vi "dfd_Check Num of Chan.vi"(7 "init in":bool, 8 "error in (no error)":errorcluster, 11 "#ch in":i32) -> (0 "error out":errorcluster, 3 "#ch out":i32, 5 "init out":bool)   [LabVIEW 2017, in "NI_DigFilter_Process.lvlib"]
uses:
  <vilib>/addons/Digital Filter Design/NI_DigFilter_Process.lvlib
  <vilib>/addons/Digital Filter Design/_Misc.llb/dfd_Error Handlers (Single).vi
  <vilib>/addons/Digital Filter Design/NI_DigFilterLicensed.lvlib
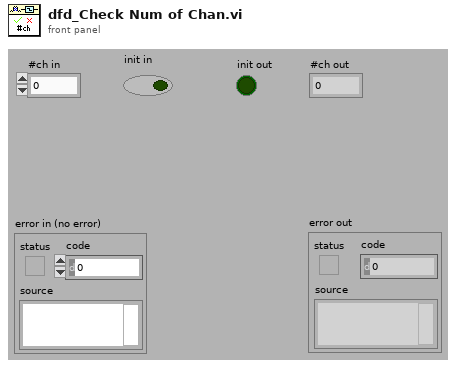
[diagram p1: front panel]
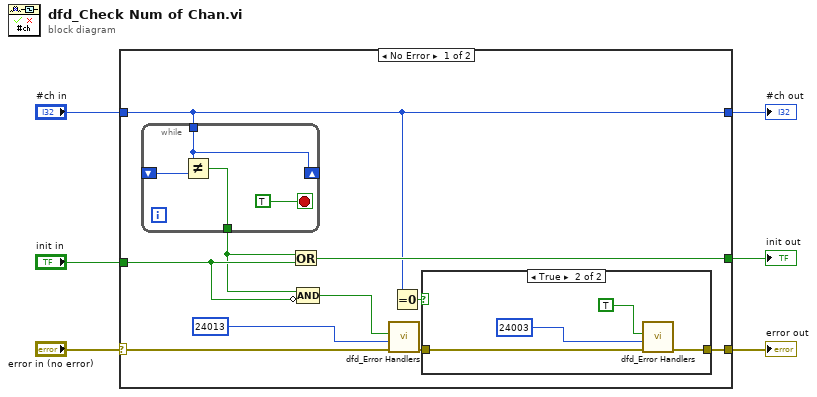
[diagram p0: block diagram]
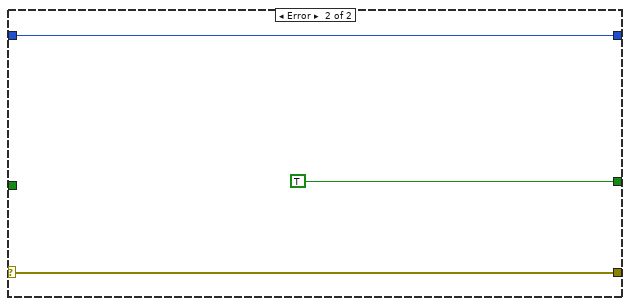
[diagram p3: hidden frame]
diagram:
  n1 = case shown="No Error" "error in (no error)" {
    selector: "error in (no error)" -> [w11 w26]
    tunnel: "init in" -> [w15 _]
    tunnel: [w16 TRUE] -> w5
    tunnel: "#ch in" -> [w10 w28]
    tunnel: [w10 w28] -> w2
    tunnel: [w8 w26] -> w1
    frame No Error {
      n2 = while {
        shift-right: [w24] -> _
        shift-left: _ -> [w25]
        tunnel: w10 -> [w24]
        tunnel: [w23] -> w14
        stop <- TRUE stop-if-true
        n3 = Not Equal?(x=w24, y=w25) -> (x != y?=w23:bool)
      }
      n4 = Or(x=w14, y=w15) -> (x .or. y?=w16:bool)
      n5 = Compound Arithmetic op=AND(w14, invert w15) -> (w13:bool)
      n6 = call-poly <vilib>:"dfd_Error Handlers.vi"("error in (no error)"=w11, "error code"=24013 ("WRN_#CH_INCONSISTENT"), "condition failed?"=w13) -> ("error out"=w7:errorcluster)  [unwired: 8 out]
      n7 = Equal To 0?(x=w10) -> (x = 0?=w9:bool)
      n8 = case shown="True" w9 {
        tunnel: w7 -> [w17 w20]
        tunnel: [w17 w19] -> w8
        frame False {
        }
        frame True {
          n9 = call-poly <vilib>:"dfd_Error Handlers.vi"("error in (no error)"=w20, "error code"=24003 ("WRN_#INPUT_ZERO"), "condition failed?"=TRUE) -> ("error out"=w19:errorcluster)  [unwired: 8 out]
        }
      }
    }
    frame Error {
    }
  }
  "error out" <- w1
  "init out" <- w5
  "#ch out" <- w2
